vi "JL_Cycle_History_ParseRecord.vi"(5 "Low Level Tries":u8=5, 7 "Error In":errorcluster, 8 "Cycle History ERD":T1={"ERD Number"=57629, "Data Type"=enum."string"} {"ERD Number" format="%.0x"}, 9 "GEA Inputs":T2={"Source"=228, "Destination"=36} {"Destination" format="%.0x"; "Source" format="%.0x"}, 10 "GEA2 Reference In":refnum<k24>) -> (0 "Error Out":errorcluster, 2 "Centauro CH Record Out":string[](array[string]), 3 "GEA2 Reference Out":refnum<k24>)   [LabVIEW 2019]
uses:
  D:/Common/LabVIEW GEA2 Toolkit/source/GEA3 DLL Source/GeaCommunication.dll
  Common/LabVIEW GEA2 Toolkit/source/GEA3 DLL Source/GeaCommunication.dll
  Common/LabVIEW GEA2 Toolkit/GEA3/type defs/Source_Destination.ctl
  Common/LabVIEW GEA2 Toolkit/GEA3/type defs/ERD Read Data In.ctl
  Common/LabVIEW GEA2 Toolkit/GEA3/library/GEA2_Toolkit.lvlib
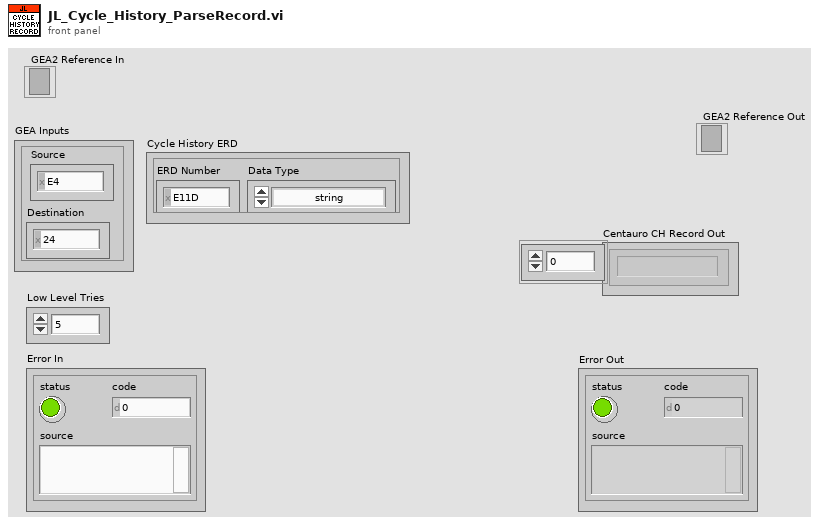
[diagram p1: front panel]
types:
  T1 = typedef "ERD Read Data In.ctl" = cluster{"ERD Number":u16, "Data Type":enum16{"string", "boolean", "uint8_t", "uint16_t", "uint32_t", "uint64_t", "int8_t", "int16_t", "int32_t", "int64_t"}}
  T2 = typedef "Source_Destination.ctl" = cluster{"Source":u8, "Destination":u8}
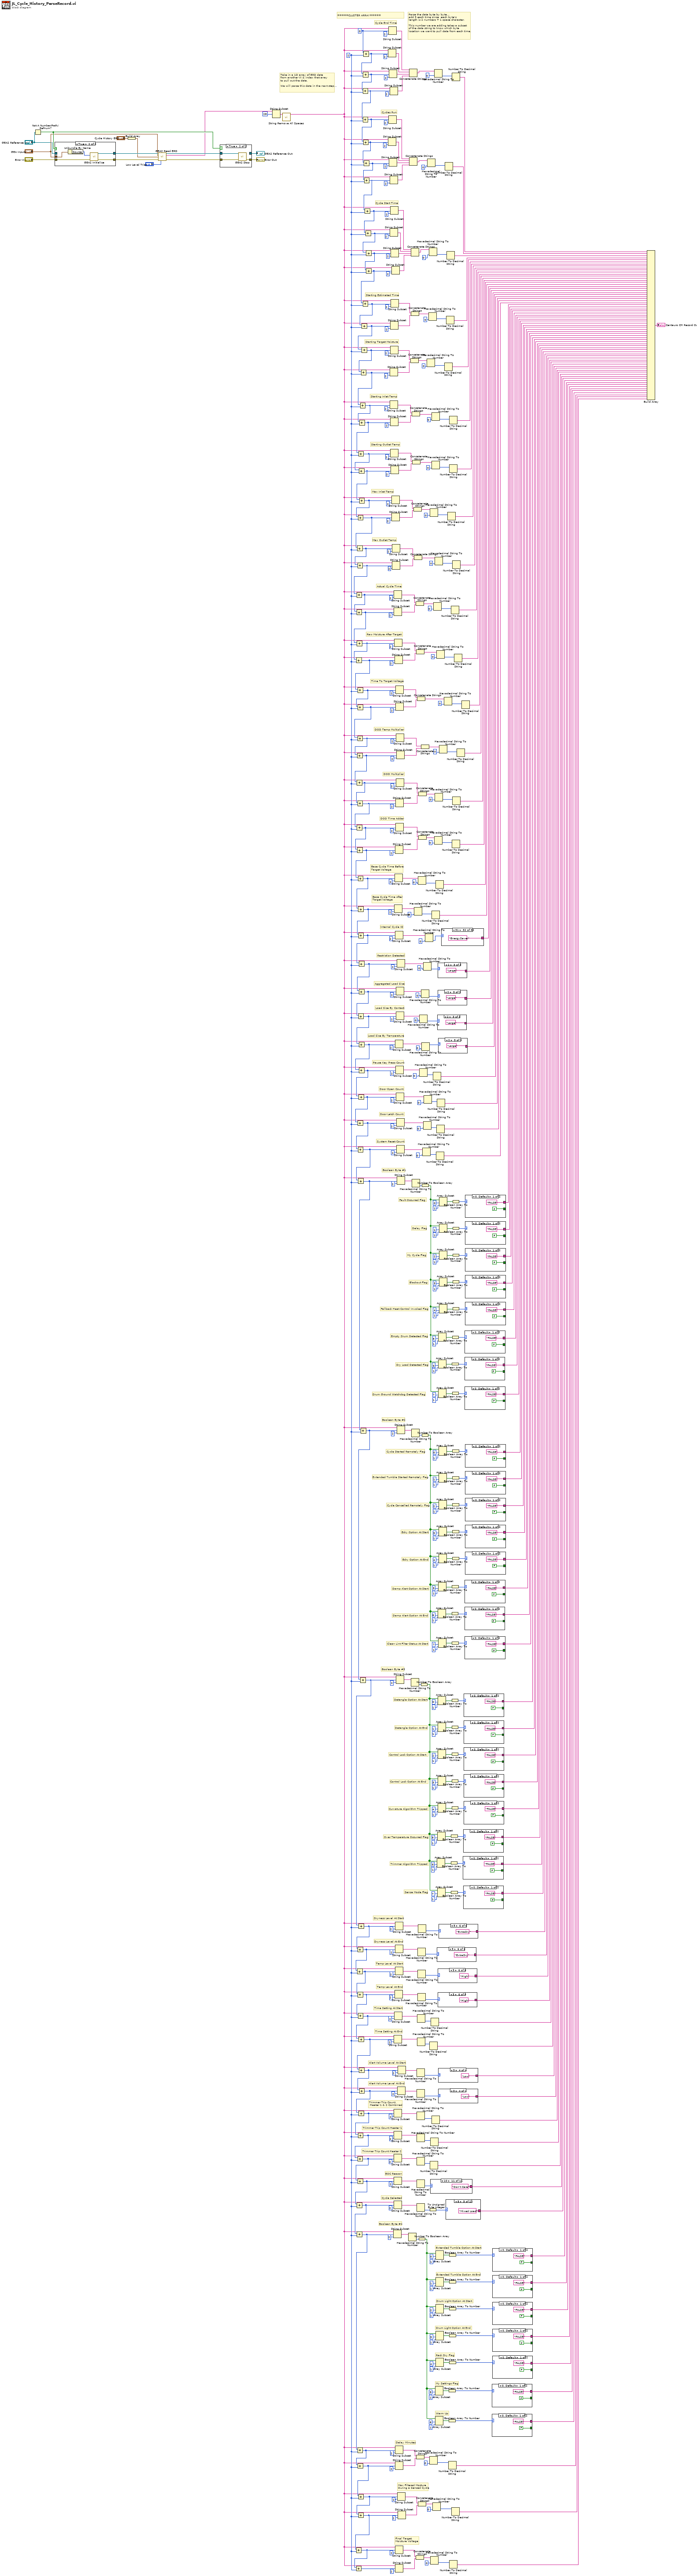
[diagram p0: block diagram]
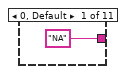
[diagram p2: hidden frame]
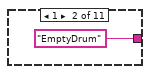
[diagram p3: hidden frame]
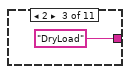
[diagram p4: hidden frame]
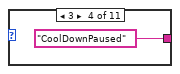
[diagram p5: hidden frame]
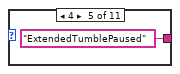
[diagram p6: hidden frame]
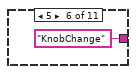
[diagram p7: hidden frame]
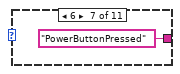
[diagram p8: hidden frame]
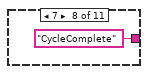
[diagram p9: hidden frame]
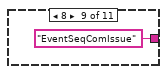
[diagram p10: hidden frame]
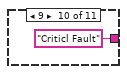
[diagram p11: hidden frame]
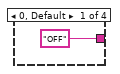
[diagram p12: hidden frame]
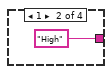
[diagram p13: hidden frame]
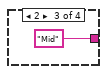
[diagram p14: hidden frame]
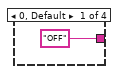
[diagram p15: hidden frame]
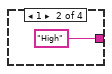
[diagram p16: hidden frame]
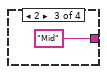
[diagram p17: hidden frame]
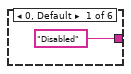
[diagram p18: hidden frame]
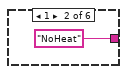
[diagram p19: hidden frame]
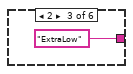
[diagram p20: hidden frame]
diagram:
  w193 = 2 ("offset (0)")
  w320 = 0 ("offset (0)")
  # "Final Target\nMoisture Voltage"
  # "Max Filtered Mosture\nDuring a Sensed Cycle"
  # "Take in a 1D array of ERD data\nfrom another VI & index that array\nto pull out the data. \n\nWe will parse this data in the next step..."
  # "Parse the data byte by byte...\nadd 3 each time since  each byte's\nlength is 2 numbers + 1 space character.\n\nThis number we are adding takes a subset\nof the data string to know which byte\nlocation we want to pull data from each time."
  # "Alert Volume Level At End"
  # "Alert Volume Level At Start"
  # "Warm Up"
  # "Delay Minutes"
  # "=====CLUSTER ARRAY====="
  # "My Settings Flag"
  # "Rack Dry Flag"
  # "Drum Light Option At End"
  # "Drum Light Option At Start"
  # "Extended Tumble Option At End"
  # "Extended Tumble Option At Start"
  # "Boolean Byte #4"
  # "Cycle Selected"
  # "EOC Reason"
  # "Trimmer Trip Count Heater 2"
  # "Trimmer Trip Count Heater 1"
  # "Trimmer Trip Count\n Heater 1 & 2 Combined"
  # "Time Setting At End"
  # "Time Setting At Start"
  # "Temp Level At End"
  # "Temp Level At Start"
  # "Dryness Level At End"
  # "Dryness Level At Start"
  # "Sense Mode Flag"
  # "Trimmer Algorithm Tripped"
  # "Over Temperature Occurred Flag"
  # "Curvature Algorithm Tripped"
  # "Control Lock Option At End"
  # "Control Lock Option At Start"
  # "Detangle Option At End"
  # "Detangle Option At Start"
  # "Boolean Byte #3"
  # "Clean Lint Filter Status At Start"
  # "Damp Alert Option At End"
  # "Damp Alert Option At Start"
  # "Edry Option At End"
  # "Edry Option At Start"
  # "Cycle Cancelled Remotely Flag"
  # "Extended Tumble Started Remotely Flag"
  # "Cycle Started Remotely Flag"
  # "Boolean Byte #2"
  # "Drum Ground Watchdog Detected Flag"
  # "Dry Load Detected Flag"
  # "Empty Drum Detected Flag"
  # "Fallback Heat Control Invoked Flag"
  # "Blackout Flag"
  # "My Cycle Flag"
  # "Delay Flag"
  # "Fault Occurred Flag"
  # "Boolean Byte #1"
  # "Door Latch Count"
  # "System Reset Count"
  # "Door Open Count"
  # "Pause Key Press Count"
  # "Load Size By Temperature"
  # "Load Size By Contact"
  # "Aggregated Load Size"
  # "Restriction Detected"
  # "Internal Cycle ID"
  # "Base Cycle Time After\nTarget Voltage"
  # "Base Cycle Time Before\nTarget Voltage"
  # "DOD Time Adder"
  # "DOD Multiplier"
  # "DOD Temp Multiplier"
  # "Time To Target Voltage"
  # "Raw Moisture After Target"
  # "Actual Cycle Time"
  # "Max Outlet Temp"
  # "Max Inlet Temp"
  # "Starting Outlet Temp"
  # "Starting Inlet Temp"
  # "Starting Target Moisture"
  # "Starting Estimated Time"
  # "Cycle Start Time"
  # "Cycles Run"
  # "Cycle End Time"
  n1 = Not A Number/Path/Refnum?(number/path/refnum="GEA2 Reference In") -> (NaN/Path/Refnum?=w190:bool)
  n2 = case shown="True" w190 {
    tunnel: "GEA Inputs" -> [_ w531]
    tunnel: "Error In" -> [w526 w530]
    tunnel: [w526 w529] -> w183
    tunnel: [w525 w528] -> w188
    tunnel: "GEA2 Reference In" -> [w525 _]
    frame False {
    }
    frame True {
      n3 = Unbundle By Name(w531) -> ("Source"=w527:u8)
      n4 = call "GEA2 Initialize.vi"("Source Address"=w527, "error in"=w530) -> ("GEA2 Reference Out"=w528:refnum<k24>, "error out"=w529:errorcluster)  [unwired: 11 in, 1 out]
    }
  }
  n5 = Build Array("Cycle History ERD") -> (w179:T1[])
  n6 = call "GEA2 Read ERD.vi"("GEA2 Reference In"=w188, "GEA Inputs"="GEA Inputs", "Read ERD List"=w179, "Error In"=w183, "Low Level Tries"="Low Level Tries") -> ("GEA2 Reference Out"=w186:refnum<k24>, "Raw Data Out"=w184:string, "Error Out"=w185:errorcluster)  [unwired: 7 in, 1 out]
  n7 = case shown="True" w190 {
    tunnel: [w532 w536] -> w191
    tunnel: [w533 _] -> w189
    tunnel: w186 -> [w533 w534]
    tunnel: w185 -> [w532 w535]
    frame False {
    }
    frame True {
      n8 = call "GEA2 Stop.vi"("GEA2 Reference In"=w534, "Error In"=w535) -> ("Error Out"=w536:errorcluster)  [unwired: 13 in]
    }
  }
  "Error Out" <- w191
  "GEA2 Reference Out" <- w189
  n9 = String Subset(string=w184, offset (0)=28) -> (substring=w177:string)  [unwired: 1 in]
  n10 = call "String Remove All Spaces.vi"("Input String"=w177) -> ("Spaces Removed"=w176:string)  [unwired: 13 in, 1 out]
  n11 = Add(x=w320, y=w193) -> (x+y=w319:i32)
  n12 = Add(x=w319, y=w193) -> (x+y=w318:i32)
  n13 = Add(x=w318, y=w193) -> (x+y=w317:i32)
  n14 = Add(x=w317, y=w193) -> (x+y=w316:i32)
  n15 = Add(x=w316, y=w193) -> (x+y=w315:i32)
  n16 = Add(x=w315, y=w193) -> (x+y=w314:i32)
  n17 = Add(x=w314, y=w193) -> (x+y=w313:i32)
  n18 = Add(x=w313, y=w193) -> (x+y=w312:i32)
  n19 = Add(x=w312, y=w193) -> (x+y=w311:i32)
  n20 = Add(x=w311, y=w193) -> (x+y=w310:i32)
  n21 = Add(x=w310, y=w193) -> (x+y=w309:i32)
  n22 = Add(x=w309, y=w193) -> (x+y=w308:i32)
  n23 = Add(x=w308, y=w193) -> (x+y=w307:i32)
  n24 = Add(x=w307, y=w193) -> (x+y=w306:i32)
  n25 = Add(x=w306, y=w193) -> (x+y=w305:i32)
  n26 = Add(x=w305, y=w193) -> (x+y=w304:i32)
  n27 = Add(x=w304, y=w193) -> (x+y=w303:i32)
  n28 = Add(x=w303, y=w193) -> (x+y=w302:i32)
  n29 = Add(x=w302, y=w193) -> (x+y=w301:i32)
  n30 = Add(x=w301, y=w193) -> (x+y=w300:i32)
  n31 = Add(x=w300, y=w193) -> (x+y=w299:i32)
  n32 = Add(x=w299, y=w193) -> (x+y=w298:i32)
  n33 = Add(x=w298, y=w193) -> (x+y=w297:i32)
  n34 = Add(x=w297, y=w193) -> (x+y=w296:i32)
  n35 = Add(x=w296, y=w193) -> (x+y=w295:i32)
  n36 = Add(x=w295, y=w193) -> (x+y=w294:i32)
  n37 = Add(x=w294, y=w193) -> (x+y=w293:i32)
  n38 = Add(x=w293, y=w193) -> (x+y=w292:i32)
  n39 = Add(x=w292, y=w193) -> (x+y=w291:i32)
  n40 = Add(x=w291, y=w193) -> (x+y=w290:i32)
  n41 = Add(x=w290, y=w193) -> (x+y=w284:i32)
  n42 = Add(x=w284, y=w193) -> (x+y=w282:i32)
  n43 = Add(x=w282, y=w193) -> (x+y=w281:i32)
  n44 = Add(x=w281, y=w193) -> (x+y=w277:i32)
  n45 = Add(x=w277, y=w193) -> (x+y=w275:i32)
  n46 = Add(x=w275, y=w193) -> (x+y=w273:i32)
  n47 = Add(x=w273, y=w193) -> (x+y=w271:i32)
  n48 = Add(x=w271, y=w193) -> (x+y=w269:i32)
  n49 = Add(x=w269, y=w193) -> (x+y=w267:i32)
  n50 = Add(x=w267, y=w193) -> (x+y=w264:i32)
  n51 = Add(x=w264, y=w193) -> (x+y=w263:i32)
  n52 = Add(x=w263, y=w193) -> (x+y=w261:i32)
  n53 = Add(x=w261, y=w193) -> (x+y=w259:i32)
  n54 = Add(x=w259, y=w193) -> (x+y=w257:i32)
  n55 = Add(x=w257, y=w193) -> (x+y=w255:i32)
  n56 = Add(x=w255, y=w193) -> (x+y=w253:i32)
  n57 = Add(x=w253, y=w193) -> (x+y=w251:i32)
  n58 = Add(x=w251, y=w193) -> (x+y=w249:i32)
  n59 = Add(x=w249, y=w193) -> (x+y=w247:i32)
  n60 = Add(x=w247, y=w193) -> (x+y=w245:i32)
  n61 = Add(x=w245, y=w193) -> (x+y=w243:i32)
  n62 = Add(x=w243, y=w193) -> (x+y=w241:i32)
  n63 = Add(x=w241, y=w193) -> (x+y=w239:i32)
  n64 = Add(x=w239, y=w193) -> (x+y=w237:i32)
  n65 = Add(x=w237, y=w193) -> (x+y=w208:i32)
  n66 = Add(x=w208, y=w193) -> (x+y=w210:i32)
  n67 = Add(x=w210, y=w193) -> (x+y=w207:i32)
  n68 = Add(x=w207, y=w193) -> (x+y=w234:i32)
  n69 = Add(x=w234, y=w193) -> (x+y=w232:i32)
  n70 = Add(x=w232, y=w193) -> (x+y=w230:i32)
  n71 = Add(x=w230, y=w193) -> (x+y=w228:i32)
  n72 = Add(x=w228, y=w193) -> (x+y=w224:i32)
  n73 = Add(x=w224, y=w193) -> (x+y=w222:i32)
  n74 = Add(x=w222, y=w193) -> (x+y=w220:i32)
  n75 = Add(x=w220, y=w193) -> (x+y=w206:i32)
  n76 = Add(x=w206, y=w193) -> (x+y=w203:i32)
  n77 = Add(x=w203, y=w193) -> (x+y=w194:i32)
  n78 = Add(x=w194, y=w193) -> (x+y=w198:i32)
  n79 = Add(x=w198, y=w193) -> (x+y=w197:i32)
  n80 = String Subset(string=w176, offset (0)=w319, length (rest)=2 ("length (rest)")) -> (substring=w519:string)
  n81 = String Subset(string=w176, offset (0)=w315, length (rest)=2 ("length (rest)")) -> (substring=w511:string)
  n82 = String Subset(string=w176, offset (0)=w320, length (rest)=2 ("length (rest)")) -> (substring=w520:string)
  n83 = String Subset(string=w176, offset (0)=w316, length (rest)=2 ("length (rest)")) -> (substring=w512:string)
  n84 = String Subset(string=w176, offset (0)=w318, length (rest)=2 ("length (rest)")) -> (substring=w518:string)
  n85 = String Subset(string=w176, offset (0)=w314, length (rest)=2 ("length (rest)")) -> (substring=w510:string)
  n86 = String Subset(string=w176, offset (0)=w317, length (rest)=2 ("length (rest)")) -> (substring=w517:string)
  n87 = String Subset(string=w176, offset (0)=w313, length (rest)=2 ("length (rest)")) -> (substring=w509:string)
  n88 = String Subset(string=w176, offset (0)=w311, length (rest)=2 ("length (rest)")) -> (substring=w503:string)
  n89 = String Subset(string=w176, offset (0)=w305, length (rest)=2 ("length (rest)")) -> (substring=w495:string)
  n90 = String Subset(string=w176, offset (0)=w304, length (rest)=2 ("length (rest)")) -> (substring=w492:string)
  n91 = String Subset(string=w176, offset (0)=w312, length (rest)=2 ("length (rest)")) -> (substring=w504:string)
  n92 = String Subset(string=w176, offset (0)=w306, length (rest)=2 ("length (rest)")) -> (substring=w496:string)
  n93 = String Subset(string=w176, offset (0)=w303, length (rest)=2 ("length (rest)")) -> (substring=w491:string)
  n94 = String Subset(string=w176, offset (0)=w307, length (rest)=2 ("length (rest)")) -> (substring=w498:string)
  n95 = String Subset(string=w176, offset (0)=w302, length (rest)=2 ("length (rest)")) -> (substring=w488:string)
  n96 = String Subset(string=w176, offset (0)=w308, length (rest)=2 ("length (rest)")) -> (substring=w499:string)
  n97 = String Subset(string=w176, offset (0)=w301, length (rest)=2 ("length (rest)")) -> (substring=w487:string)
  n98 = String Subset(string=w176, offset (0)=w310, length (rest)=2 ("length (rest)")) -> (substring=w502:string)
  n99 = String Subset(string=w176, offset (0)=w309, length (rest)=2 ("length (rest)")) -> (substring=w501:string)
  n100 = String Subset(string=w176, offset (0)=w300, length (rest)=2 ("length (rest)")) -> (substring=w484:string)
  n101 = String Subset(string=w176, offset (0)=w299, length (rest)=2 ("length (rest)")) -> (substring=w483:string)
  n102 = String Subset(string=w176, offset (0)=w298, length (rest)=2 ("length (rest)")) -> (substring=w480:string)
  n103 = String Subset(string=w176, offset (0)=w297, length (rest)=2 ("length (rest)")) -> (substring=w479:string)
  n104 = String Subset(string=w176, offset (0)=w222, length (rest)=2 ("length (rest)")) -> (substring=w346:string)
  n105 = String Subset(string=w176, offset (0)=w296, length (rest)=2 ("length (rest)")) -> (substring=w476:string)
  n106 = String Subset(string=w176, offset (0)=w230, length (rest)=2 ("length (rest)")) -> (substring=w351:string)
  n107 = String Subset(string=w176, offset (0)=w224, length (rest)=2 ("length (rest)")) -> (substring=w349:string)
  n108 = String Subset(string=w176, offset (0)=w295, length (rest)=2 ("length (rest)")) -> (substring=w475:string)
  n109 = String Subset(string=w176, offset (0)=w208, length (rest)=2 ("length (rest)")) -> (substring=w354:string)
  n110 = String Subset(string=w176, offset (0)=w234, length (rest)=2 ("length (rest)")) -> (substring=w353:string)
  n111 = String Subset(string=w176, offset (0)=w232, length (rest)=2 ("length (rest)")) -> (substring=w352:string)
  n112 = String Subset(string=w176, offset (0)=w228, length (rest)=2 ("length (rest)")) -> (substring=w350:string)
  n113 = String Subset(string=w176, offset (0)=w294, length (rest)=2 ("length (rest)")) -> (substring=w472:string)
  n114 = String Subset(string=w176, offset (0)=w271, length (rest)=2 ("length (rest)")) -> (substring=w107:string)
  n115 = String Subset(string=w176, offset (0)=w237, length (rest)=2 ("length (rest)")) -> (substring=w355:string)
  n116 = String Subset(string=w176, offset (0)=w293, length (rest)=2 ("length (rest)")) -> (substring=w471:string)
  n117 = String Subset(string=w176, offset (0)=w273, length (rest)=2 ("length (rest)")) -> (substring=w114:string)
  n118 = String Subset(string=w176, offset (0)=w239, length (rest)=2 ("length (rest)")) -> (substring=w356:string)
  n119 = String Subset(string=w176, offset (0)=w269, length (rest)=2 ("length (rest)")) -> (substring=w99:string)
  n120 = String Subset(string=w176, offset (0)=w243, length (rest)=2 ("length (rest)")) -> (substring=w358:string)
  n121 = String Subset(string=w176, offset (0)=w241, length (rest)=2 ("length (rest)")) -> (substring=w357:string)
  n122 = String Subset(string=w176, offset (0)=w198, length (rest)=2 ("length (rest)")) -> (substring=w196:string)
  n123 = String Subset(string=w176, offset (0)=w275, length (rest)=2 ("length (rest)")) -> (substring=w278:string)
  n124 = String Subset(string=w176, offset (0)=w261, length (rest)=2 ("length (rest)")) -> (substring=w91:string)
  n125 = String Subset(string=w176, offset (0)=w245, length (rest)=2 ("length (rest)")) -> (substring=w359:string)
  n126 = String Subset(string=w176, offset (0)=w220, length (rest)=2 ("length (rest)")) -> (substring=w226:string)
  n127 = String Subset(string=w176, offset (0)=w206, length (rest)=2 ("length (rest)")) -> (substring=w225:string)
  n128 = String Subset(string=w176, offset (0)=w197, length (rest)=2 ("length (rest)")) -> (substring=w195:string)
  n129 = String Subset(string=w176, offset (0)=w292, length (rest)=2 ("length (rest)")) -> (substring=w468:string)
  n130 = String Subset(string=w176, offset (0)=w281, length (rest)=2 ("length (rest)")) -> (substring=w288:string)
  n131 = String Subset(string=w176, offset (0)=w291, length (rest)=2 ("length (rest)")) -> (substring=w467:string)
  n132 = String Subset(string=w176, offset (0)=w277, length (rest)=2 ("length (rest)")) -> (substring=w279:string)
  n133 = String Subset(string=w176, offset (0)=w259, length (rest)=2 ("length (rest)")) -> (substring=w87:string)
  n134 = String Subset(string=w176, offset (0)=w290, length (rest)=2 ("length (rest)")) -> (substring=w175:string)
  n135 = String Subset(string=w176, offset (0)=w282, length (rest)=2 ("length (rest)")) -> (substring=w289:string)
  n136 = String Subset(string=w176, offset (0)=w264, length (rest)=2 ("length (rest)")) -> (substring=w102:string)
  n137 = String Subset(string=w176, offset (0)=w263, length (rest)=2 ("length (rest)")) -> (substring=w96:string)
  n138 = String Subset(string=w176, offset (0)=w257, length (rest)=2 ("length (rest)")) -> (substring=w79:string)
  n139 = String Subset(string=w176, offset (0)=w247, length (rest)=2 ("length (rest)")) -> (substring=w394:string)
  n140 = String Subset(string=w176, offset (0)=w284, length (rest)=2 ("length (rest)")) -> (substring=w174:string)
  n141 = String Subset(string=w176, offset (0)=w255, length (rest)=2 ("length (rest)")) -> (substring=w76:string)
  n142 = String Subset(string=w176, offset (0)=w253, length (rest)=2 ("length (rest)")) -> (substring=w73:string)
  n143 = String Subset(string=w176, offset (0)=w267, length (rest)=2 ("length (rest)")) -> (substring=w104:string)
  n144 = String Subset(string=w176, offset (0)=w249, length (rest)=2 ("length (rest)")) -> (substring=w429:string)
  n145 = String Subset(string=w176, offset (0)=w251, length (rest)=2 ("length (rest)")) -> (substring=w464:string)
  n146 = String Subset(string=w176, offset (0)=w207, length (rest)=2 ("length (rest)")) -> (substring=w212:string)
  n147 = String Subset(string=w176, offset (0)=w203, length (rest)=2 ("length (rest)")) -> (substring=w202:string)
  n148 = String Subset(string=w176, offset (0)=w210, length (rest)=2 ("length (rest)")) -> (substring=w213:string)
  n149 = String Subset(string=w176, offset (0)=w194, length (rest)=2 ("length (rest)")) -> (substring=w201:string)
  n150 = Hexadecimal String To Number(string=w346) -> (number=w345:u32)  [unwired: 2 in, 1 out]
  n151 = Concatenate Strings(w520, w519, w518, w517) -> (w173:string)
  n152 = Concatenate Strings(w512, w511, w510, w509) -> (w169:string)
  n153 = Concatenate Strings(w496, w495) -> (w155:string)
  n154 = Concatenate Strings(w504, w503, w502, w501) -> (w166:string)
  n155 = Concatenate Strings(w499, w498) -> (w163:string)
  n156 = Hexadecimal String To Number(string=w394) -> (number=w393:u32)  [unwired: 2 in, 1 out]
  n157 = Hexadecimal String To Number(string=w429) -> (number=w428:u32)  [unwired: 2 in, 1 out]
  n158 = Concatenate Strings(w492, w491) -> (w151:string)
  n159 = Hexadecimal String To Number(string=w464) -> (number=w463:u32)  [unwired: 2 in, 1 out]
  n160 = Concatenate Strings(w488, w487) -> (w147:string)
  n161 = Concatenate Strings(w484, w483) -> (w144:string)
  n162 = Concatenate Strings(w480, w479) -> (w139:string)
  n163 = Hexadecimal String To Number(string=w107, default (0uL)=u8 0) -> (number=w108:u8)  [unwired: 1 in, 1 out]
  n164 = Concatenate Strings(w476, w475) -> (w135:string)
  n165 = Concatenate Strings(w196, w195) -> (w6:string)
  n166 = Concatenate Strings(w472, w471) -> (w131:string)
  n167 = Concatenate Strings(w226, w225) -> (w13:string)
  n168 = Hexadecimal String To Number(string=w213) -> (number=w33:u32)  [unwired: 2 in, 1 out]
  n169 = Hexadecimal String To Number(string=w212) -> (number=w31:u32)  [unwired: 2 in, 1 out]
  n170 = Hexadecimal String To Number(string=w353) -> (number=w29:u32)  [unwired: 2 in, 1 out]
  n171 = Hexadecimal String To Number(string=w352) -> (number=w27:u32)  [unwired: 2 in, 1 out]
  n172 = Hexadecimal String To Number(string=w351) -> (number=w25:u32)  [unwired: 2 in, 1 out]
  n173 = Hexadecimal String To Number(string=w350) -> (number=w23:u32)  [unwired: 2 in, 1 out]
  n174 = Hexadecimal String To Number(string=w349) -> (number=w348:u32)  [unwired: 2 in, 1 out]
  n175 = Hexadecimal String To Number(string=w354) -> (number=w35:u32)  [unwired: 2 in, 1 out]
  n176 = Concatenate Strings(w468, w467) -> (w127:string)
  n177 = Hexadecimal String To Number(string=w355) -> (number=w37:u32)  [unwired: 2 in, 1 out]
  n178 = Hexadecimal String To Number(string=w356) -> (number=w39:u32)  [unwired: 2 in, 1 out]
  n179 = Hexadecimal String To Number(string=w358) -> (number=w43:u32)  [unwired: 2 in, 1 out]
  n180 = Hexadecimal String To Number(string=w357) -> (number=w41:u32)  [unwired: 2 in, 1 out]
  n181 = Hexadecimal String To Number(string=w114, default (0uL)=u8 0) -> (number=w115:u8)  [unwired: 1 in, 1 out]
  n182 = Hexadecimal String To Number(string=w359) -> (number=w45:u32)  [unwired: 2 in, 1 out]
  n183 = Number To Boolean Array(number=w345) -> (Boolean array=w214:bool[])
  n184 = Concatenate Strings(w202, w201) -> (w8:string)
  n185 = Concatenate Strings(w289, w288) -> (w119:string)
  n186 = Concatenate Strings(w279, w278) -> (w116:string)
  n187 = Hexadecimal String To Number(string=w87, default (0uL)=u8 0) -> (number=w89:u8)  [unwired: 1 in, 1 out]
  n188 = Hexadecimal String To Number(string=w96, default (0uL)=u8 0) -> (number=w93:u8)  [unwired: 1 in, 1 out]
  n189 = Number To Boolean Array(number=w393) -> (Boolean array=w360:bool[])
  n190 = Number To Boolean Array(number=w428) -> (Boolean array=w395:bool[])
  n191 = Concatenate Strings(w175, w174) -> (w123:string)
  n192 = Hexadecimal String To Number(string=w102, default (0uL)=u8 0) -> (number=w94:u8)  [unwired: 1 in, 1 out]
  n193 = Number To Boolean Array(number=w463) -> (Boolean array=w430:bool[])
  n194 = Hexadecimal String To Number(string=w91, default (0uL)=u8 0) -> (offset past number=w90:i32)  [unwired: 1 in, 1 out]
  n195 = Hexadecimal String To Number(string=w73, default (0uL)=u8 0) -> (number=w74:u8)  [unwired: 1 in, 1 out]
  n196 = Hexadecimal String To Number(string=w104, default (0uL)=u8 0) -> (number=w95:u8)  [unwired: 1 in, 1 out]
  n197 = Hexadecimal String To Number(string=w76, default (0uL)=u8 0) -> (number=w78:u8)  [unwired: 1 in, 1 out]
  n198 = Hexadecimal String To Number(string=w79, default (0uL)=u8 0) -> (number=w80:u8)  [unwired: 1 in, 1 out]
  n199 = Hexadecimal String To Number(string=w99, default (0uL)=u8 0) -> (number=w98:u8)  [unwired: 1 in, 1 out]
  n200 = Hexadecimal String To Number(string=w155, default (0uL)=u16 0) -> (number=w156:u16)  [unwired: 1 in, 1 out]
  n201 = Hexadecimal String To Number(string=w169, default (0uL)=u32 0) -> (number=w170:u32)  [unwired: 1 in, 1 out]
  n202 = Hexadecimal String To Number(string=w163, default (0uL)=u16 0) -> (number=w164:u16)  [unwired: 1 in, 1 out]
  n203 = Hexadecimal String To Number(string=w166, default (0uL)=u32 0) -> (number=w167:u32)  [unwired: 1 in, 1 out]
  n204 = To Unsigned Byte Integer(number=w348) -> (unsigned 8bit integer=w347:u8)
  n205 = Number To Decimal String(number=w35) -> (decimal integer string=w34:string)  [unwired: 1 in]
  n206 = Hexadecimal String To Number(string=w13, default (0uL)=u16 0 ("default (0 U32)")) -> (number=w12:u16)  [unwired: 1 in, 1 out]
  n207 = Hexadecimal String To Number(string=w144, default (0uL)=u16 0) -> (number=w145:u16)  [unwired: 1 in, 1 out]
  n208 = Number To Decimal String(number=w25) -> (decimal integer string=w24:string)  [unwired: 1 in]
  n209 = Number To Decimal String(number=w27) -> (decimal integer string=w26:string)  [unwired: 1 in]
  n210 = case shown="10" w23 {
    tunnel: ["NA" "EmptyDrum" "DryLoad" "CoolDownPaused" "ExtendedTumblePaused" "KnobChange" "PowerButtonPressed" "CycleComplete" "EventSeqComIssue" "Criticl Fault" "Don't Care"] -> w22
    frame 0, Default {
    }
    frame 1 {
    }
    frame 2 {
    }
    frame 3 {
    }
    frame 4 {
    }
    frame 5 {
    }
    frame 6 {
    }
    frame 7 {
    }
    frame 8 {
    }
    frame 9 {
    }
    frame 10 {
    }
  }
  n211 = Hexadecimal String To Number(string=w6, default (0uL)=u16 0 ("default (0 U32)")) -> (number=w5:u16)  [unwired: 1 in, 1 out]
  n212 = Number To Decimal String(number=w37) -> (decimal integer string=w36:string)  [unwired: 1 in]
  n213 = Number To Decimal String(number=w108) -> (decimal integer string=w106:string)  [unwired: 1 in]
  n214 = Number To Decimal String(number=w29) -> (decimal integer string=w28:string)  [unwired: 1 in]
  n215 = Hexadecimal String To Number(string=w151, default (0uL)=u16 0) -> (number=w153:u16)  [unwired: 1 in, 1 out]
  n216 = Hexadecimal String To Number(string=w147, default (0uL)=u16 0) -> (number=w148:u16)  [unwired: 1 in, 1 out]
  n217 = Hexadecimal String To Number(string=w8, default (0uL)=u16 0 ("default (0 U32)")) -> (number=w9:u16)  [unwired: 1 in, 1 out]
  n218 = Number To Decimal String(number=w89) -> (decimal integer string=w82:string)  [unwired: 1 in]
  n219 = Hexadecimal String To Number(string=w135, default (0uL)=u16 0) -> (number=w137:u16)  [unwired: 1 in, 1 out]
  n220 = Hexadecimal String To Number(string=w173, default (0uL)=u32 0) -> (number=w172:u32)  [unwired: 1 in, 1 out]
  n221 = Hexadecimal String To Number(string=w116, default (0uL)=u16 0) -> (number=w117:u16)  [unwired: 1 in, 1 out]
  n222 = Hexadecimal String To Number(string=w119, default (0uL)=u16 0) -> (number=w121:u16)  [unwired: 1 in, 1 out]
  n223 = Hexadecimal String To Number(string=w139, default (0uL)=u16 0) -> (number=w140:u16)  [unwired: 1 in, 1 out]
  n224 = Array Subset(array=w214, index=5, length=1) -> (w321:bool[])
  n225 = Array Subset(array=w214, index=6, length=1) -> (w215:bool[])
  n226 = Number To Decimal String(number=w115) -> (decimal integer string=w110:string)  [unwired: 1 in]
  n227 = Array Subset(array=w214, index=0, length=1) -> (w329:bool[])
  n228 = Array Subset(array=w214, index=1, length=1) -> (w328:bool[])
  n229 = Array Subset(array=w214, index=2, length=1) -> (w327:bool[])
  n230 = Array Subset(array=w214, index=3, length=1) -> (w326:bool[])
  n231 = Array Subset(array=w214, index=4, length=1) -> (w325:bool[])
  n232 = Number To Decimal String(number=w74) -> (decimal integer string=w70:string)  [unwired: 1 in]
  n233 = Hexadecimal String To Number(string=w131, default (0uL)=u16 0) -> (number=w132:u16)  [unwired: 1 in, 1 out]
  n234 = Number To Decimal String(number=w78) -> (decimal integer string=w71:string)  [unwired: 1 in]
  n235 = case shown="5" w43 {
    tunnel: ["Disabled" "Damp" "LessDry" "Dry" "MoreDry" "ExtraDry"] -> w42
    frame 0, Default {
    }
    frame 1 {
    }
    frame 2 {
    }
    frame 3 {
    }
    frame 4 {
    }
    frame 5 {
    }
  }
  n236 = Number To Decimal String(number=w80) -> (decimal integer string=w72:string)  [unwired: 1 in]
  n237 = Array Subset(array=w360, index=6, length=1) -> (w365:bool[])
  n238 = case shown="2" w93 {
    tunnel: ["Undefined" "Small" "Large"] -> w84
    frame 0, Default {
    }
    frame 1 {
    }
    frame 2 {
    }
  }
  n239 = Array Subset(array=w360, index=5, length=1) -> (w369:bool[])
  n240 = Array Subset(array=w360, index=7, length=1) -> (w361:bool[])
  n241 = case shown="2" w94 {
    tunnel: ["Undefined" "Small" "Large"] -> w85
    frame 0, Default {
    }
    frame 1 {
    }
    frame 2 {
    }
  }
  n242 = case shown="5" w41 {
    tunnel: ["Disabled" "NoHeat" "ExtraLow" "Low" "Medium" "High"] -> w40
    frame 0, Default {
    }
    frame 1 {
    }
    frame 2 {
    }
    frame 3 {
    }
    frame 4 {
    }
    frame 5 {
    }
  }
  n243 = case shown="5" w39 {
    tunnel: ["Disabled" "NoHeat" "ExtraLow" "Low" "Medium" "High"] -> w38
    frame 0, Default {
    }
    frame 1 {
    }
    frame 2 {
    }
    frame 3 {
    }
    frame 4 {
    }
    frame 5 {
    }
  }
  n244 = case shown="2" w95 {
    tunnel: ["Undefined" "Small" "Large"] -> w86
    frame 0, Default {
    }
    frame 1 {
    }
    frame 2 {
    }
  }
  n245 = Array Subset(array=w395, index=6, length=1) -> (w400:bool[])
  n246 = Array Subset(array=w360, index=0, length=1) -> (w377:bool[])
  n247 = Array Subset(array=w360, index=1, length=1) -> (w376:bool[])
  n248 = Array Subset(array=w360, index=2, length=1) -> (w375:bool[])
  n249 = Array Subset(array=w360, index=3, length=1) -> (w374:bool[])
  n250 = Array Subset(array=w360, index=4, length=1) -> (w373:bool[])
  n251 = Array Subset(array=w430, index=6, length=1) -> (w435:bool[])
  n252 = Array Subset(array=w395, index=5, length=1) -> (w404:bool[])
  n253 = Array Subset(array=w395, index=7, length=1) -> (w396:bool[])
  n254 = case shown="2" w90 {
    tunnel: ["Undefined" "Small" "Large"] -> w83
    frame 0, Default {
    }
    frame 1 {
    }
    frame 2 {
    }
  }
  n255 = Array Subset(array=w430, index=5, length=1) -> (w439:bool[])
  n256 = Array Subset(array=w430, index=7, length=1) -> (w431:bool[])
  n257 = case shown="3" w33 {
    tunnel: ["OFF" "High" "Mid" "Low"] -> w32
    frame 0, Default {
    }
    frame 1 {
    }
    frame 2 {
    }
    frame 3 {
    }
  }
  n258 = case shown="3" w31 {
    tunnel: ["OFF" "High" "Mid" "Low"] -> w30
    frame 0, Default {
    }
    frame 1 {
    }
    frame 2 {
    }
    frame 3 {
    }
  }
  n259 = Array Subset(array=w395, index=0, length=1) -> (w412:bool[])
  n260 = Array Subset(array=w395, index=1, length=1) -> (w411:bool[])
  n261 = Array Subset(array=w395, index=2, length=1) -> (w410:bool[])
  n262 = Array Subset(array=w395, index=3, length=1) -> (w409:bool[])
  n263 = Array Subset(array=w395, index=4, length=1) -> (w408:bool[])
  n264 = case shown="5" w45 {
    tunnel: ["Disabled" "Damp" "LessDry" "Dry" "MoreDry" "ExtraDry"] -> w44
    frame 0, Default {
    }
    frame 1 {
    }
    frame 2 {
    }
    frame 3 {
    }
    frame 4 {
    }
    frame 5 {
    }
  }
  n265 = Hexadecimal String To Number(string=w123, default (0uL)=u16 0) -> (number=w124:u16)  [unwired: 1 in, 1 out]
  n266 = Array Subset(array=w430, index=0, length=1) -> (w447:bool[])
  n267 = Array Subset(array=w430, index=1, length=1) -> (w446:bool[])
  n268 = Array Subset(array=w430, index=2, length=1) -> (w445:bool[])
  n269 = Array Subset(array=w430, index=3, length=1) -> (w444:bool[])
  n270 = Array Subset(array=w430, index=4, length=1) -> (w443:bool[])
  n271 = case shown="31" w98 {
    tunnel: ["Unmapped" "MixedLoad" "Casuals" "Delicates" "SpeedDry" "Jeans" "TimedDry" "Warmup" "AirFluff" "SteamDewrinkle" "SteamDewrinkle" "SanitizeDry" "BulkyItems" "TowelsSheets" "Cottons" "CasualsLessDry" "CasualsMoreDry" "CottonsLessDry" "CottonsOptimumDry" "CottonsMoreDry" "DelicatesLessDry" "DelicatesMoreDry" "TimeDry1" "TimeDry2" "TimeDry3" "TimeDry4" "TimeDry5" "TimeDry6" "ActiveWear" "DeWrinkle" "QuickDry" "EnergySaver"] -> w97
    frame 0, Default {
    }
    frame 1 {
    }
    frame 2 {
    }
    frame 3 {
    }
    frame 4 {
    }
    frame 5 {
    }
    frame 6 {
    }
    frame 7 {
    }
    frame 8 {
    }
    frame 9 {
    }
    frame 10 {
    }
    frame 11 {
    }
    frame 12 {
    }
    frame 13 {
    }
    frame 14 {
    }
    frame 15 {
    }
    frame 16 {
    }
    frame 17 {
    }
    frame 18 {
    }
    frame 19 {
    }
    frame 20 {
    }
    frame 21 {
    }
    frame 22 {
    }
    frame 23 {
    }
    frame 24 {
    }
    frame 25 {
    }
    frame 26 {
    }
    frame 27 {
    }
    frame 28 {
    }
    frame 29 {
    }
    frame 30 {
    }
    frame 31 {
    }
  }
  n272 = Hexadecimal String To Number(string=w127, default (0uL)=u16 0) -> (number=w129:u16)  [unwired: 1 in, 1 out]
  n273 = Number To Decimal String(number=w156) -> (decimal integer string=w154:string)  [unwired: 1 in]
  n274 = Number To Decimal String(number=w170) -> (decimal integer string=w168:string)  [unwired: 1 in]
  n275 = case shown="8" w347 {
    tunnel: ["Not Defined" "Bulky Items" "Sanitize" "Towels/Sheets" "Mixed Load" "Jeans" "Delicates" "Cottons" "Easy Care" "Active Wear" "Timed Dry" "DeWrinkle" "Quick/Air Fluff" "Steam Refresh" "Steam Dewrinkle" "Speed Dry" "Mixed" "Quick dry" "Casuals" "Warm up" "Energy Saver"] -> w21
    frame 0, Default {
    }
    frame 4 {
    }
    frame 5 {
    }
    frame 6 {
    }
    frame 8 {
    }
    frame 11 {
    }
    frame 13 {
    }
    frame 128 {
    }
    frame 129 {
    }
    frame 130 {
    }
    frame 131 {
    }
    frame 132 {
    }
    frame 133 {
    }
    frame 134 {
    }
    frame 135 {
    }
    frame 136 {
    }
    frame 137 {
    }
    frame 138 {
    }
    frame 139 {
    }
    frame 140 {
    }
    frame 141 {
    }
  }
  n276 = Number To Decimal String(number=w164) -> (decimal integer string=w158:string)  [unwired: 1 in]
  n277 = Number To Decimal String(number=w167) -> (decimal integer string=w165:string)  [unwired: 1 in]
  n278 = Number To Decimal String(number=w145) -> (decimal integer string=w142:string)  [unwired: 1 in]
  n279 = Boolean Array To Number(Boolean array=w321) -> (number=w324:u32)
  n280 = Boolean Array To Number(Boolean array=w215) -> (number=w218:u32)
  n281 = Number To Decimal String(number=w12) -> (decimal integer string=w4:string)  [unwired: 1 in]
  n282 = Boolean Array To Number(Boolean array=w329) -> (number=w344:u32)
  n283 = Boolean Array To Number(Boolean array=w328) -> (number=w343:u32)
  n284 = Boolean Array To Number(Boolean array=w327) -> (number=w342:u32)
  n285 = Boolean Array To Number(Boolean array=w326) -> (number=w341:u32)
  n286 = Boolean Array To Number(Boolean array=w325) -> (number=w340:u32)
  n287 = Number To Decimal String(number=w153) -> (decimal integer string=w150:string)  [unwired: 1 in]
  n288 = Number To Decimal String(number=w148) -> (decimal integer string=w146:string)  [unwired: 1 in]
  n289 = Number To Decimal String(number=w5) -> (decimal integer string=w2:string)  [unwired: 1 in]
  n290 = Boolean Array To Number(Boolean array=w365) -> (number=w368:u32)
  n291 = Boolean Array To Number(Boolean array=w369) -> (number=w372:u32)
  n292 = Boolean Array To Number(Boolean array=w361) -> (number=w364:u32)
  n293 = Number To Decimal String(number=w137) -> (decimal integer string=w134:string)  [unwired: 1 in]
  n294 = Boolean Array To Number(Boolean array=w400) -> (number=w403:u32)
  n295 = Boolean Array To Number(Boolean array=w377) -> (number=w392:u32)
  n296 = Boolean Array To Number(Boolean array=w376) -> (number=w391:u32)
  n297 = Boolean Array To Number(Boolean array=w375) -> (number=w390:u32)
  n298 = Boolean Array To Number(Boolean array=w374) -> (number=w389:u32)
  n299 = Boolean Array To Number(Boolean array=w373) -> (number=w388:u32)
  n300 = Boolean Array To Number(Boolean array=w435) -> (number=w438:u32)
  n301 = Boolean Array To Number(Boolean array=w404) -> (number=w407:u32)
  n302 = Boolean Array To Number(Boolean array=w396) -> (number=w399:u32)
  n303 = Boolean Array To Number(Boolean array=w439) -> (number=w442:u32)
  n304 = Boolean Array To Number(Boolean array=w431) -> (number=w434:u32)
  n305 = Number To Decimal String(number=w9) -> (decimal integer string=w3:string)  [unwired: 1 in]
  n306 = Boolean Array To Number(Boolean array=w412) -> (number=w427:u32)
  n307 = Boolean Array To Number(Boolean array=w411) -> (number=w426:u32)
  n308 = Boolean Array To Number(Boolean array=w410) -> (number=w425:u32)
  n309 = Boolean Array To Number(Boolean array=w409) -> (number=w424:u32)
  n310 = Boolean Array To Number(Boolean array=w408) -> (number=w423:u32)
  n311 = Number To Decimal String(number=w172) -> (decimal integer string=w171:string)  [unwired: 1 in]
  n312 = Number To Decimal String(number=w117) -> (decimal integer string=w111:string)  [unwired: 1 in]
  n313 = Boolean Array To Number(Boolean array=w447) -> (number=w462:u32)
  n314 = Boolean Array To Number(Boolean array=w446) -> (number=w461:u32)
  n315 = Boolean Array To Number(Boolean array=w445) -> (number=w460:u32)
  n316 = Boolean Array To Number(Boolean array=w444) -> (number=w459:u32)
  n317 = Boolean Array To Number(Boolean array=w443) -> (number=w458:u32)
  n318 = Number To Decimal String(number=w121) -> (decimal integer string=w112:string)  [unwired: 1 in]
  n319 = Number To Decimal String(number=w140) -> (decimal integer string=w138:string)  [unwired: 1 in]
  n320 = Number To Decimal String(number=w132) -> (decimal integer string=w130:string)  [unwired: 1 in]
  n321 = Number To Decimal String(number=w124) -> (decimal integer string=w122:string)  [unwired: 1 in]
  n322 = Number To Decimal String(number=w129) -> (decimal integer string=w126:string)  [unwired: 1 in]
  n323 = case shown="0, Default" w368 {
    tunnel: [FALSE TRUE] -> _
    tunnel: ["FALSE" "TRUE"] -> w47
    frame 0, Default {
    }
    frame 1 {
    }
  }
  n324 = case shown="0, Default" w372 {
    tunnel: [FALSE TRUE] -> _
    tunnel: ["FALSE" "TRUE"] -> w48
    frame 0, Default {
    }
    frame 1 {
    }
  }
  n325 = case shown="0, Default" w364 {
    tunnel: [FALSE TRUE] -> _
    tunnel: ["FALSE" "TRUE"] -> w46
    frame 0, Default {
    }
    frame 1 {
    }
  }
  n326 = case shown="0, Default" w392 {
    tunnel: [FALSE TRUE] -> _
    tunnel: ["FALSE" "TRUE"] -> w53
    frame 0, Default {
    }
    frame 1 {
    }
  }
  n327 = case shown="0, Default" w391 {
    tunnel: [FALSE TRUE] -> _
    tunnel: ["FALSE" "TRUE"] -> w52
    frame 0, Default {
    }
    frame 1 {
    }
  }
  n328 = case shown="0, Default" w390 {
    tunnel: [FALSE TRUE] -> _
    tunnel: ["FALSE" "TRUE"] -> w51
    frame 0, Default {
    }
    frame 1 {
    }
  }
  n329 = case shown="0, Default" w389 {
    tunnel: [FALSE TRUE] -> _
    tunnel: ["FALSE" "TRUE"] -> w50
    frame 0, Default {
    }
    frame 1 {
    }
  }
  n330 = case shown="0, Default" w388 {
    tunnel: [FALSE TRUE] -> _
    tunnel: ["FALSE" "TRUE"] -> w49
    frame 0, Default {
    }
    frame 1 {
    }
  }
  n331 = case shown="0, Default" w438 {
    tunnel: [FALSE TRUE] -> _
    tunnel: ["FALSE" "TRUE"] -> w63
    frame 0, Default {
    }
    frame 1 {
    }
  }
  n332 = case shown="0, Default" w403 {
    tunnel: [FALSE TRUE] -> _
    tunnel: ["FALSE" "TRUE"] -> w55
    frame 0, Default {
    }
    frame 1 {
    }
  }
  n333 = case shown="0, Default" w442 {
    tunnel: [FALSE TRUE] -> _
    tunnel: ["FALSE" "TRUE"] -> w64
    frame 0, Default {
    }
    frame 1 {
    }
  }
  n334 = case shown="0, Default" w434 {
    tunnel: [FALSE TRUE] -> _
    tunnel: ["FALSE" "TRUE"] -> w62
    frame 0, Default {
    }
    frame 1 {
    }
  }
  n335 = case shown="0, Default" w407 {
    tunnel: [FALSE TRUE] -> _
    tunnel: ["FALSE" "TRUE"] -> w56
    frame 0, Default {
    }
    frame 1 {
    }
  }
  n336 = case shown="0, Default" w399 {
    tunnel: [FALSE TRUE] -> _
    tunnel: ["FALSE" "TRUE"] -> w54
    frame 0, Default {
    }
    frame 1 {
    }
  }
  n337 = case shown="0, Default" w462 {
    tunnel: [FALSE TRUE] -> _
    tunnel: ["FALSE" "TRUE"] -> w69
    frame 0, Default {
    }
    frame 1 {
    }
  }
  n338 = case shown="0, Default" w461 {
    tunnel: [FALSE TRUE] -> _
    tunnel: ["FALSE" "TRUE"] -> w68
    frame 0, Default {
    }
    frame 1 {
    }
  }
  n339 = case shown="0, Default" w460 {
    tunnel: [FALSE TRUE] -> _
    tunnel: ["FALSE" "TRUE"] -> w67
    frame 0, Default {
    }
    frame 1 {
    }
  }
  n340 = case shown="0, Default" w459 {
    tunnel: [FALSE TRUE] -> _
    tunnel: ["FALSE" "TRUE"] -> w66
    frame 0, Default {
    }
    frame 1 {
    }
  }
  n341 = case shown="0, Default" w458 {
    tunnel: [FALSE TRUE] -> _
    tunnel: ["FALSE" "TRUE"] -> w65
    frame 0, Default {
    }
    frame 1 {
    }
  }
  n342 = case shown="0, Default" w427 {
    tunnel: [FALSE TRUE] -> _
    tunnel: ["FALSE" "TRUE"] -> w61
    frame 0, Default {
    }
    frame 1 {
    }
  }
  n343 = case shown="0, Default" w426 {
    tunnel: [FALSE TRUE] -> _
    tunnel: ["FALSE" "TRUE"] -> w60
    frame 0, Default {
    }
    frame 1 {
    }
  }
  n344 = case shown="0, Default" w425 {
    tunnel: [FALSE TRUE] -> _
    tunnel: ["FALSE" "TRUE"] -> w59
    frame 0, Default {
    }
    frame 1 {
    }
  }
  n345 = case shown="0, Default" w424 {
    tunnel: [FALSE TRUE] -> _
    tunnel: ["FALSE" "TRUE"] -> w58
    frame 0, Default {
    }
    frame 1 {
    }
  }
  n346 = case shown="0, Default" w423 {
    tunnel: [FALSE TRUE] -> _
    tunnel: ["FALSE" "TRUE"] -> w57
    frame 0, Default {
    }
    frame 1 {
    }
  }
  n347 = case shown="0, Default" w324 {
    tunnel: [FALSE TRUE] -> _
    tunnel: ["FALSE" "TRUE"] -> w15
    frame 0, Default {
    }
    frame 1 {
    }
  }
  n348 = case shown="0, Default" w218 {
    tunnel: [FALSE TRUE] -> _
    tunnel: ["FALSE" "TRUE"] -> w14
    frame 0, Default {
    }
    frame 1 {
    }
  }
  n349 = case shown="0, Default" w344 {
    tunnel: [FALSE TRUE] -> _
    tunnel: ["FALSE" "TRUE"] -> w20
    frame 0, Default {
    }
    frame 1 {
    }
  }
  n350 = case shown="0, Default" w343 {
    tunnel: [FALSE TRUE] -> _
    tunnel: ["FALSE" "TRUE"] -> w19
    frame 0, Default {
    }
    frame 1 {
    }
  }
  n351 = case shown="0, Default" w342 {
    tunnel: [FALSE TRUE] -> _
    tunnel: ["FALSE" "TRUE"] -> w18
    frame 0, Default {
    }
    frame 1 {
    }
  }
  n352 = case shown="0, Default" w341 {
    tunnel: [FALSE TRUE] -> _
    tunnel: ["FALSE" "TRUE"] -> w17
    frame 0, Default {
    }
    frame 1 {
    }
  }
  n353 = case shown="0, Default" w340 {
    tunnel: [FALSE TRUE] -> _
    tunnel: ["FALSE" "TRUE"] -> w16
    frame 0, Default {
    }
    frame 1 {
    }
  }
  n354 = Build Array(w171, w168, w165, w158, w154, w150, w146, w142, w138, w134, w130, w126, w122, w112, w111, w110, w106, w97, w86, w85, w84, w83, w82, w72, w71, w70, w69, w68, w67, w66, w65, w64, w63, w62, w61, w60, w59, w58, w57, w56, w55, w54, w53, w52, w51, w50, w49, w48, w47, w46, w44, w42, w40, w38, w36, w34, w32, w30, w28, w26, w24, w22, w21, w20, w19, w18, w17, w16, w15, w14, w4, w3, w2) -> (→"Centauro CH Record Out":string[])
